vi "_RT Process Set Table.vi"(8 "Error In":errorcluster, 9 "Data":string, 11 "Command":T1) -> (0 "Error Out":errorcluster)   [LabVIEW 2015]
uses:
  Type/_RT Command.ctl
  _RT Global.vi
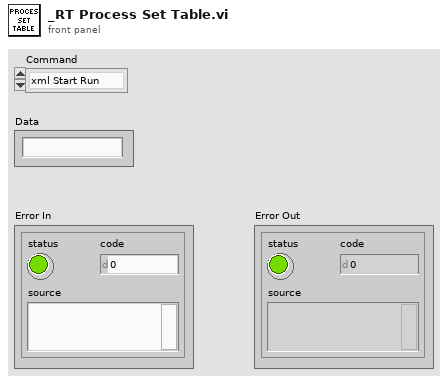
[diagram p1: front panel]
types:
  T1 = typedef "_RT Command.ctl" = enum16{"xml Start Run", "xml Start Actual Run", "xml Stop Run", "xml Runtime Update", "xml Get Status", "xml Get Table", "xml Set Table", "xml Get Configuration", "xml System Status", "xml Set LC Input Logic", "xml Get Data", "xml Get Info", "Start", "StartActualRun", "Stop", "Runtime Update", "Get Data", "Get Info", "Get Status", "Get Param", "Get Config", "Get Table", "Read ADC", "Set Oscillator", "Update Config", "Update Table", "Set All Pol", "Set Pol and DC", "Set Max Mass", "Toggle RP", "Toggle EL", "Set PIC", "Initialize Turbo", "Send Turbo Comm", "Close Turbo", "P1", "P2", "P3", "Send Serial", "Set LC Out", "Get LC In", "Read VAC", "Test Table", "Toggle Power", "Get Startup", "Set Startup", "Get ADC Table", "Set ADC Table", "Get Brief Status", "Get Detail Status", "Auxiliary Update", "Set CC Logics", "Set CC Input Logics", "Ignore Error", "invalid"}
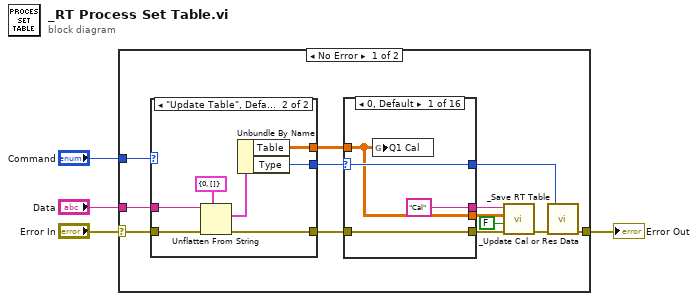
[diagram p0: block diagram]
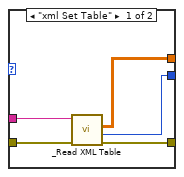
[diagram p2: hidden frame]
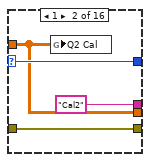
[diagram p3: hidden frame]
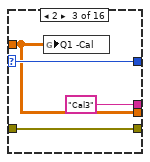
[diagram p4: hidden frame]
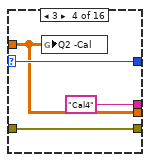
[diagram p5: hidden frame]
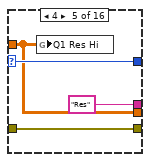
[diagram p6: hidden frame]
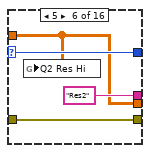
[diagram p7: hidden frame]
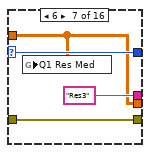
[diagram p8: hidden frame]
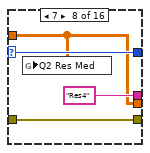
[diagram p9: hidden frame]
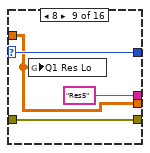
[diagram p10: hidden frame]
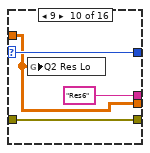
[diagram p11: hidden frame]
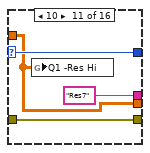
[diagram p12: hidden frame]
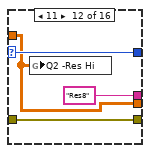
[diagram p13: hidden frame]
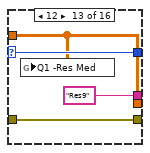
[diagram p14: hidden frame]
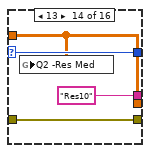
[diagram p15: hidden frame]
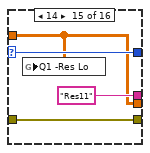
[diagram p16: hidden frame]
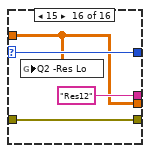
[diagram p17: hidden frame]
diagram:
  n1 = case shown="No Error" "Error In" {
    selector: "Error In" -> [w13 w94]
    tunnel: [w15 w94] -> w4
    tunnel: "Data" -> [w14 _]
    tunnel: "Command" -> [w12 _]
    frame No Error {
      n2 = case shown="\"Update Table\", Default" w12 {
        tunnel: w14 -> [w22 w29]
        tunnel: [w20 w24] -> w7
        tunnel: w13 -> [w21 w25]
        tunnel: [w19 w26] -> w9
        tunnel: [w18 w23] -> w10
        frame "xml Set Table" {
          n3 = call "_Read XML Table.vi"("error in"=w21, "XML String"=w22) -> ("error out"=w20:errorcluster, "Table Type"=w18:i32, "Table (2D-DBL)"=w19:dbl[][])  [unwired: 3 out]
        }
        frame "Update Table", Default {
          n4 = Unflatten From String(type=cluster{"Type":u16, "Table":dbl[][]} {"Type"=0, "Table"=[]} ("Calibration"), binary string=w29, error in (no error)=w25) -> (value=w27:cluster{"Type":u16, "Table":dbl[][]}, error out=w24:errorcluster)  [unwired: 3 out]
          n5 = Unbundle By Name(w27) -> ("Table"=w26:dbl[][], "Type"=w23:u16)
        }
      }
      n6 = case shown="0, Default" w10 {
        selector: w10 -> [w32 w36 w40 w44 w48 w52 w56 w60 w64 w68 w72 w76 w80 w84 w88 w92]
        tunnel: ["Cal" ("key") "Cal2" ("key") "Cal3" ("key") "Cal4" ("key") "Res" ("key") "Res2" ("key") "Res3" ("key") "Res4" ("key") "Res5" ("key") "Res6" ("key") "Res7" ("key") "Res8" ("key") "Res9" ("key") "Res10" ("key") "Res11" ("key") "Res12" ("key")] -> w17
        tunnel: [w32 w36 w40 w44 w48 w52 w56 w60 w64 w68 w72 w76 w80 w84 w88 w92] -> w11
        tunnel: w9 -> [w30 w34 w38 w42 w46 w50 w54 w58 w62 w66 w70 w74 w78 w82 w86 w90]
        tunnel: [w31 w35 w39 w43 w47 w51 w55 w59 w63 w67 w71 w75 w79 w83 w87 w91] -> w8
        tunnel: w7 -> [w31 w35 w39 w43 w47 w51 w55 w59 w63 w67 w71 w75 w79 w83 w87 w91]
        tunnel: [w30 w34 w38 w42 w46 w50 w54 w58 w62 w66 w70 w74 w78 w82 w86 w90] -> w6
        frame 0, Default {
          n7 = global write "_RT Global.vi" "Q1 Cal"(w30) -> ()
        }
        frame 1 {
          n8 = global write "_RT Global.vi" "Q2 Cal"(w34) -> ()
        }
        frame 2 {
          n9 = global write "_RT Global.vi" "Q1 -Cal"(w38) -> ()
        }
        frame 3 {
          n10 = global write "_RT Global.vi" "Q2 -Cal"(w42) -> ()
        }
        frame 4 {
          n11 = global write "_RT Global.vi" "Q1 Res Hi"(w46) -> ()
        }
        frame 5 {
          n12 = global write "_RT Global.vi" "Q2 Res Hi"(w50) -> ()
        }
        frame 6 {
          n13 = global write "_RT Global.vi" "Q1 Res Med"(w54) -> ()
        }
        frame 7 {
          n14 = global write "_RT Global.vi" "Q2 Res Med"(w58) -> ()
        }
        frame 8 {
          n15 = global write "_RT Global.vi" "Q1 Res Lo"(w62) -> ()
        }
        frame 9 {
          n16 = global write "_RT Global.vi" "Q2 Res Lo"(w66) -> ()
        }
        frame 10 {
          n17 = global write "_RT Global.vi" "Q1 -Res Hi"(w70) -> ()
        }
        frame 11 {
          n18 = global write "_RT Global.vi" "Q2 -Res Hi"(w74) -> ()
        }
        frame 12 {
          n19 = global write "_RT Global.vi" "Q1 -Res Med"(w78) -> ()
        }
        frame 13 {
          n20 = global write "_RT Global.vi" "Q2 -Res Med"(w82) -> ()
        }
        frame 14 {
          n21 = global write "_RT Global.vi" "Q1 -Res Lo"(w86) -> ()
        }
        frame 15 {
          n22 = global write "_RT Global.vi" "Q2 -Res Lo"(w90) -> ()
        }
      }
      n23 = call "_Save RT Table.vi"("error in (no error)"=w8, "Simulation"=FALSE, "Table"=w6, "key"=w17) -> ("error out"=w16:errorcluster)  [unwired: 3 out]
      n24 = call "_Update Cal or Res Data.vi"("error in (no error)"=w16, "Table Type"=w11) -> ("error out"=w15:errorcluster)  [unwired: 1 in, 4 out]
    }
    frame Error {
    }
  }
  "Error Out" <- w4
